vi "VISA Locking.vi"() -> ()   [LabVIEW 2023]
doc: "This examples demonstrates VISA locking. The VISA locking mechanism enforces arbitration of accesses to resources on an individual basis. Typically, the programmer will use lock and unlock around critical pieces of code. If a session locks a resource, operations invoked by other sessions are returned with a locked error. Shared locks may also be used although these aren't demonstrated here.\n\nThis VI opens two sessions to the same instrument and locks the first session. The first session then writes the String to Write to the instrument and reads a response of the desired length. The second session attempts to do the same task but will not succeed until the first session is unlocked, which will allow the second session to perform its read/write operation successfully.\n\nTypically, the two different sessions would be in separate VIs or applications, rather than in the same VI as this example demonstrates."
panel:
  in  "Release Lock":bool
  out "response from second session":string
  out "response from first session":string
  in  "string to write":string="*IDN?"
  in  "timeout for second session (ms)":u32=10000
  in  "VISA Resource 2":refnum<visa-resource-name>
  in  "VISA Resource 1":refnum<visa-resource-name>
  # "Overview: Demonstrates the use of the VISA functions to execute VISA locking.\nRequirements: NI-VISA Driver\nInstructions:\n1. Ensure the resources specified in the VISA Resource 1 and VISA Resource 2 controls are to the same device.\n2. Run the VI.\n3. Click the Release Lock button to release the VISA lock on the first session so the second session can complete."
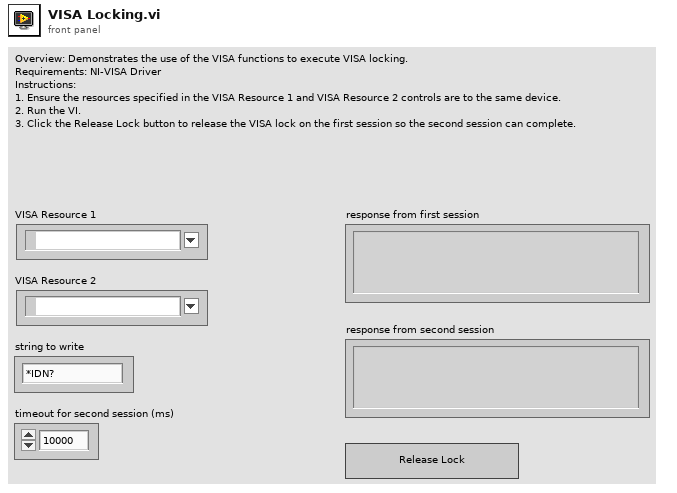
[diagram p1: front panel]
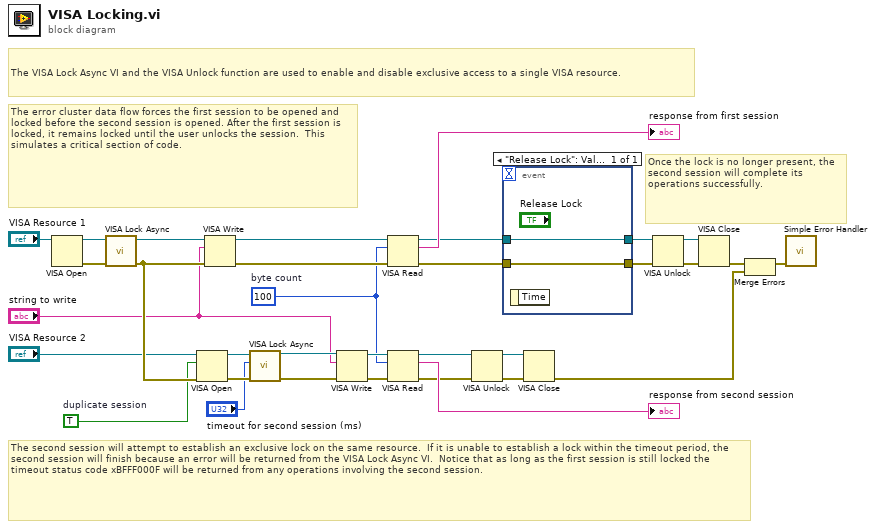
[diagram p0: block diagram]
diagram:
  w9 = u32 100  # byte count
  w11 = TRUE  # duplicate session
  # "The VISA Lock Async VI and the VISA Unlock function are used to enable and disable exclusive access to a single VISA resource."
  # "Once the lock is no longer present, the second session will complete its operations successfully."
  # "The second session will attempt to establish an exclusive lock on the same resource.  If it is unable to establish a lock within the timeout period, the second session will finish because an error will be returned from the VISA Lock Async VI.  Notice that as long as the first session is still locked the timeout status code xBFFF000F will be returned from any operations involving the second session."
  # "The error cluster data flow forces the first session to be opened and locked before the second session is opened. After the first session is locked, it remains locked until the user unlocks the session.  This simulates a critical section of code."
  n1 = VISA Open(VISA resource name="VISA Resource 1") -> (VISA resource name=w17:refnum<visa-resource-name>, error out=w18:errorcluster)  [unwired: 1 in, 3 out]
  n2 = call <vilib>:"VISA Lock Async.vi"("error in (no error)"=w18, "VISA resource name"=w17) -> ("error out"=w13:errorcluster, "VISA resource name out"=w33:refnum<visa-resource-name>)  [unwired: 1 in, 7 out]
  n3 = VISA Open(duplicate session (F)=w11, error in (no error)=w13, VISA resource name="VISA Resource 2") -> (VISA resource name=w14:refnum<visa-resource-name>, error out=w15:errorcluster)  [unwired: 2 out]
  n4 = VISA Write(VISA resource name=w33, write buffer="string to write", error in (no error)=w13) -> (VISA resource name out=w32:refnum<visa-resource-name>, error out=w31:errorcluster)  [unwired: 1 out]
  n5 = call <vilib>:"VISA Lock Async.vi"("error in (no error)"=w15, "timeout (0)"="timeout for second session (ms)", "VISA resource name"=w14) -> ("error out"=w25:errorcluster, "VISA resource name out"=w24:refnum<visa-resource-name>)  [unwired: 7 out]
  n6 = VISA Write(VISA resource name=w24, write buffer="string to write", error in (no error)=w25) -> (VISA resource name out=w27:refnum<visa-resource-name>, error out=w23:errorcluster)  [unwired: 1 out]
  n7 = VISA Read(VISA resource name=w32, byte count=w9, error in (no error)=w31) -> (VISA resource name out=w7:refnum<visa-resource-name>, read buffer=→"response from first session":string, error out=w5:errorcluster)  [unwired: 1 out]
  n8 = VISA Read(VISA resource name=w27, byte count=w9, error in (no error)=w23) -> (VISA resource name out=w22:refnum<visa-resource-name>, read buffer=→"response from second session":string, error out=w19:errorcluster)  [unwired: 1 out]
  n9 = VISA Unlock(8:w19, 11:w22) -> (0:w20:errorcluster, 3:w21:refnum<visa-resource-name>)
  n10 = event shown="[0] \"Release Lock\": Value Change" {
    selector: _ -> [_]
    dyn-events: _ -> [_]
    timeout: _ -> [_]
    tunnel: w7 -> [w35]
    tunnel: [w35] -> w6
    tunnel: w5 -> [w34]
    tunnel: [w34] -> w4
    event "Release Lock": Value Change {
      n11 = event-data() -> ()  [unwired: 1 in, 1 out]
    }
  }
  n12 = VISA Close(VISA resource name=w21, error in (no error)=w20) -> (error out=w1:errorcluster)
  n13 = VISA Unlock(8:w4, 11:w6) -> (0:w28:errorcluster, 3:w29:refnum<visa-resource-name>)
  n14 = VISA Close(VISA resource name=w29, error in (no error)=w28) -> (error out=w3:errorcluster)
  n15 = Merge Errors(w3, w1) -> (w2:errorcluster)
  n16 = call <vilib>:"Simple Error Handler.vi"("error in (no error)"=w2) -> ()  [unwired: 1 in, 8 out]
